vi "InitImg.vi"(8 "error in (no error)":errorcluster, 11 "EpiWrapper in":refnum<class "EpiWrapper.lvclass">) -> (0 "error out":errorcluster, 3 "EpiWrapper out":refnum<class "EpiWrapper.lvclass">)   [LabVIEW 2012, in "EpiWrapper.lvclass"]
uses:
  EpiWrapper.lvclass
  EpiWrapper.lvclass/EpiWrapper.ctl
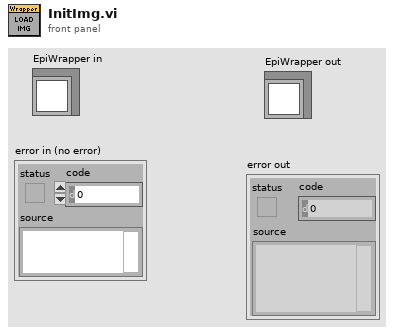
[diagram p1: front panel]
types:
  T1 = typedef "LVBoundsTypeDef.ctl" = cluster{"Width":u32, "Height":u32}
  T2 = typedef "imagedata.ctl" = cluster{"image type":i32, "image depth":i32, "image":u8[], "mask":u8[], "colors":u32[], "Rectangle":cluster{"left":i16, "top":i16, "right":i16, "bottom":i16}}
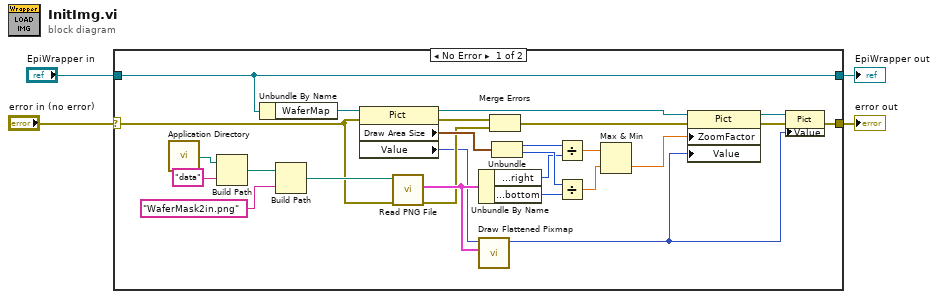
[diagram p0: block diagram]
diagram:
  n1 = case shown="No Error" "error in (no error)" {
    selector: "error in (no error)" -> [w8 w32]
    tunnel: [w10 w32] -> w3
    tunnel: [w7 w31] -> w1
    tunnel: "EpiWrapper in" -> [w7 w31]
    frame No Error {
      n2 = call <vilib>:"Application Directory.vi"() -> ("Application Directory"=w30:path)
      n3 = Build Path(base path=w30, name or relative path="data") -> (appended path=w13:path)
      n4 = Unbundle By Name(w7) -> ("WaferMap"=w9:refnum<vi>)
      n5 = Build Path(base path=w13, name or relative path="WaferMask2in.png") -> (appended path=w11:path)
      n6 = property class="Pict"(reference=w9, error in=w8) -> (reference out=w21:refnum<vi>, error out=w18:errorcluster, "Draw Area Size"=w22:T1, "Value"=w5:picture)
      n7 = call <vilib>:"Read PNG File.vi"("error in (no error)"=w8, "path to PNG file"=w11) -> ("error out"=w19:errorcluster, "image data"=w29:T2)  [unwired: 7 in, 1 out]
      n8 = Unbundle By Name(w29) -> ("Rectangle.right"=w25:i16, "Rectangle.bottom"=w26:i16)
      n9 = call <vilib>:"Draw Flattened Pixmap.vi"("image data"=w29, "picture"=w5) -> ("new picture"=w6:picture)  [unwired: 7 in]
      n10 = Merge Errors(w18, w19) -> (w17:errorcluster)
      n11 = Unbundle(w22) -> ("Width"=w28:u32, "Height"=w27:u32)
      n12 = Divide(x=w28, y=w25) -> (x/y=w24:dbl)
      n13 = Divide(x=w27, y=w26) -> (x/y=w23:dbl)
      n14 = Max & Min(x=w24, y=w23) -> (min(x,y)=w20:dbl)  [unwired: 1 out]
      n15 = property class="Pict"(reference=w21, error in=w17, "ZoomFactor"=w20, "Value"=w6) -> (reference out=w16:refnum<vi>, error out=w15:errorcluster)
      n16 = property class="Pict"(reference=w16, error in=w15, "Value"=w6) -> (error out=w10:errorcluster)  [unwired: 1 out]
    }
    frame Error {
    }
  }
  "error out" <- w3
  "EpiWrapper out" <- w1
